vi "SetDough.vi"(8 "error in (no error)":errorcluster, 10 "Dough":string, 11 "object in":refnum<class "Pizza(Product).lvclass">) -> (0 "error out":errorcluster, 3 "object out":refnum<class "Pizza(Product).lvclass">)   [LabVIEW 2014, in "Pizza(Product).lvclass"]
uses:
  Pizza(Product).lvclass
  Pizza(Product).lvclass/Pizza(Product).ctl
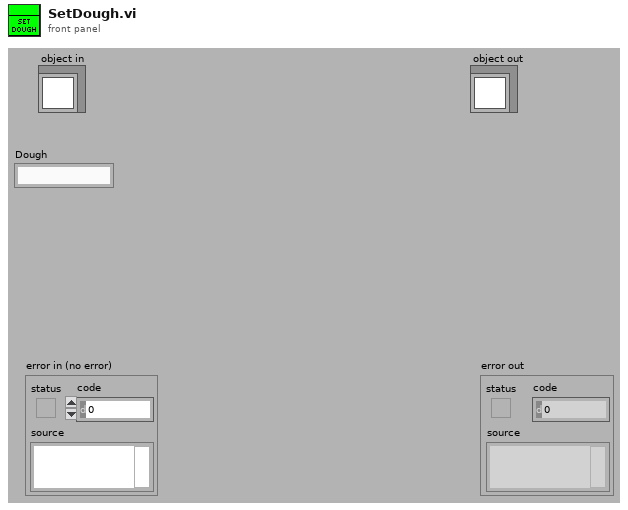
[diagram p1: front panel]
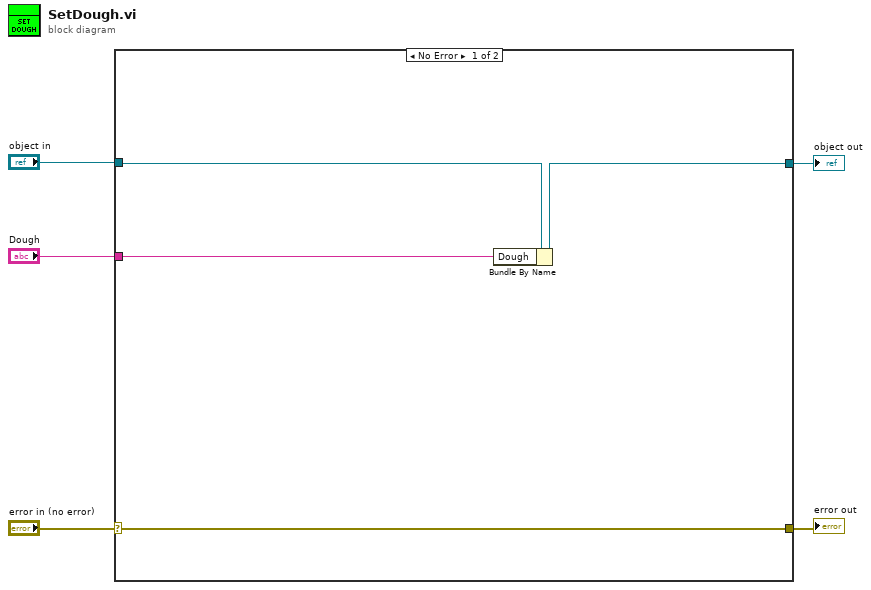
[diagram p0: block diagram]
diagram:
  n1 = case shown="No Error" "error in (no error)" {
    selector: "error in (no error)" -> [w9 w11]
    tunnel: [w9 w11] -> w4
    tunnel: [w7 w10] -> w2
    tunnel: "object in" -> [w8 w10]
    tunnel: "Dough" -> [w6 _]
    frame No Error {
      n2 = Bundle By Name(cluster=w8, "Dough"=w6) -> (w7:refnum<class "Pizza(Product).lvclass">)
    }
    frame Error {
    }
  }
  "error out" <- w4
  "object out" <- w2
